vi "Volume entry-Initialise z-step control.vi"(8 "error in (no error)":errorcluster, 11 "# of planes":i32) -> (0 "error out":errorcluster)   [LabVIEW 2017]
uses:
  ROI Entry screen/Globals/gl_Volume Entry UI globals.vi
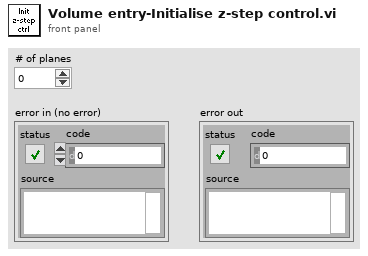
[diagram p1: front panel]
types:
  T1 = typedef "Volume entry ctrl refs cluster.ctl" = cluster{"Z-step (planes)":refnum<vi>, "Volume":refnum<vi>, "Dual Rectangle":refnum<vi>, "Zoom":refnum<vi>, "Z-plane 1":refnum<vi>, "Z-plane 2":refnum<vi>, "ZplaneIndex (zero based)":refnum<vi>}
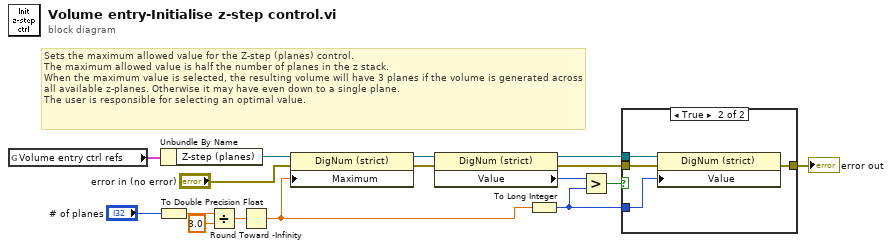
[diagram p0: block diagram]
diagram:
  # "Sets the maximum allowed value for the Z-step (planes) control.\nThe maximum allowed value is half the number of planes in the z stack.\nWhen the maximum value is selected, the resulting volume will have 3 planes if the volume is generated across all available z-planes. Otherwise it may have even down to a single plane.\nThe user is responsible for selecting an optimal value."
  n1 = global read "gl_Volume Entry UI globals.vi" "Volume entry ctrl refs"() -> (w1:T1)
  n2 = To Double Precision Float(number="# of planes") -> (double precision float=w4:dbl)
  n3 = Unbundle By Name(w1) -> ("Z-step (planes)"=w12:refnum<vi>)
  n4 = Divide(x=w4, y=3.0) -> (x/y=w5:dbl)
  n5 = Round Toward -Infinity(1:w5) -> (0:w6:dbl)
  n6 = property on="Property Node" class="DigNum (strict)"(reference=w12, error in="error in (no error)", "Maximum"=w6) -> (reference out=w8:refnum<vi>, error out=w13:errorcluster)
  n7 = property on="Property Node" class="DigNum (strict)"(reference=w8, error in=w13) -> (reference out=w9:refnum<vi>, error out=w14:errorcluster, "Value"=w7:i32)
  n8 = To Long Integer(number=w6) -> (32bit integer=w11:i32)
  n9 = Greater?(x=w7, y=w11) -> (0:w10:bool)
  n10 = case shown="True" w10 {
    tunnel: w9 -> [_ w21]
    tunnel: w11 -> [_ w20]
    tunnel: w14 -> [w17 w19]
    tunnel: [w17 w18] -> w15
    frame False {
    }
    frame True {
      n11 = property on="Property Node" class="DigNum (strict)"(reference=w21, error in=w19, "Value"=w20) -> (error out=w18:errorcluster)  [unwired: 1 out]
    }
  }
  "error out" <- w15
